vi "VI Scripting with Structures - Flat Sequence Structure.vi"   [LabVIEW 2023]
doc: "This example contains sample code demonstrating common VI Scripting navigational tasks relating to Flat Sequence Structures."
panel:
  # "Overview: Illustrates several FlatSequence properties and methods used for inspecting and modifying Flat Sequence Structures with VI Scripting.\nInstructions:\nOpen the block diagram of this VI to see several examples of properties and methods related to Flat Sequence Structures and VI Scripting.\n\nNote: Browse the diagram of this example to learn about VI Scripting concepts. This example is not meant to be run."
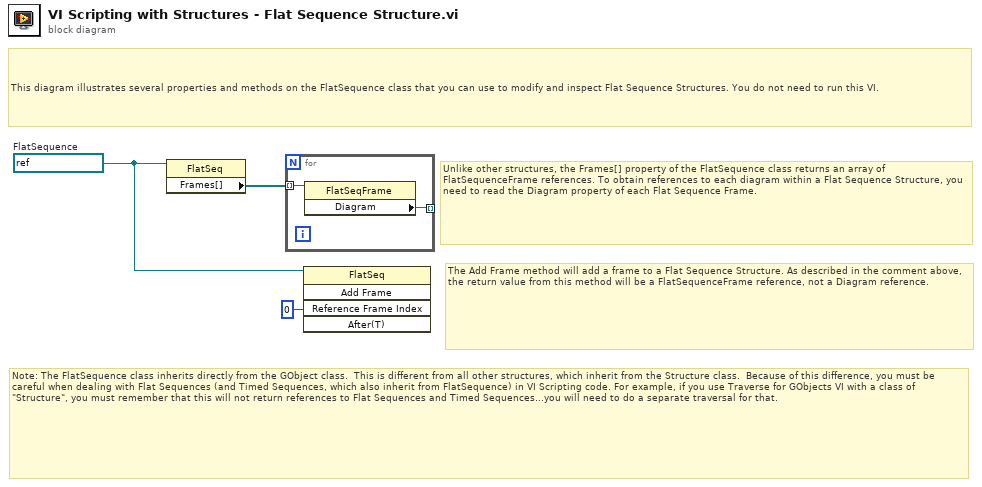
[diagram p0: block diagram]
diagram:
  w3 = refnum<vi> refnum  # FlatSequence
  # "Note: The FlatSequence class inherits directly from the GObject class.  This is different from all other structures, which inherit from the Structure class.  Because of this difference, you must be careful when dealing with Flat Sequences (and Timed Sequences, which also inherit from FlatSequence) in VI Scripting code. For example, if you use Traverse for GObjects VI with a class of \"Structure\", you must remember that this will not return references to Flat Sequences and Timed Sequences...you will need to do a separate traversal for that."
  # "The Add Frame method will add a frame to a Flat Sequence Structure. As described in the comment above, the return value from this method will be a FlatSequenceFrame reference, not a Diagram reference."
  # "This diagram illustrates several properties and methods on the FlatSequence class that you can use to modify and inspect Flat Sequence Structures. You do not need to run this VI."
  # "Unlike other structures, the Frames[] property of the FlatSequence class returns an array of FlatSequenceFrame references. To obtain references to each diagram within a Flat Sequence Structure, you need to read the Diagram property of each Flat Sequence Frame."
  n1 = property class="FlatSeq"(reference=w3) -> ("Frames[]"=w1:refnum<vi>[])  [unwired: 1 in, 2 out]
  n2 = for {
    tunnel: w1 -> [w5] mode=indexing
    tunnel: [w4] -> _ mode=indexing
    n3 = property class="FlatSeqFrame"(reference=w5) -> ("Diagram"=w4:refnum<vi>)  [unwired: 1 in, 2 out]
  }
  n4 = invoke class="FlatSeq" method="Add Frame"(reference=w3, "Reference Frame Index"=u32 0) -> ()  [unwired: 3 in, 5 out]
